vi "Read Bytes.vi"(8 "Error In":errorcluster) -> (0 "Error Out":errorcluster)   [LabVIEW 2017, in "Tests.lvlib" / "Reader.lvlib"]
uses:
  Reader.lvlib
  src/LabPack/Public/Reader/Reader.lvclass/Reader.ctl
  src/LabPack/Public/Reader/Private/Read Bytes by Value.vi
  src/LabPack/Public/Reader/Private/Handle Error.vi
  src/LabPack/Public/Reader/Public/Status/Read Status.vi
  src/LabPack/Public/Reader/Public/Status/Read Status Message.vi
  src/LabPack/Public/Reader/Public/Status/Read Is Error.vi
  src/LabPack/Public/Reader/Private/Begin Bin by Value.vi
  src/LabPack/Public/Utility/Status Code.vi
  <vilib>/Utility/error.llb/Error Cluster From Error Code.vi
  src/LabPack/Public/Reader/Private/End Bin by Value.vi
  <vilib>/addons/_JKI Toolkits/Caraya/classes/Test/Test.lvclass
  <vilib>/addons/_JKI Toolkits/Caraya/classes/Assert/Assert.lvclass
  src/LabPack/Public/Reader/Reader.lvclass
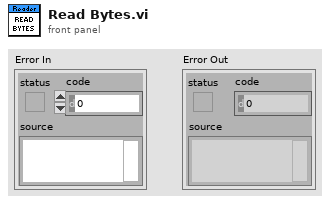
[diagram p1: front panel]
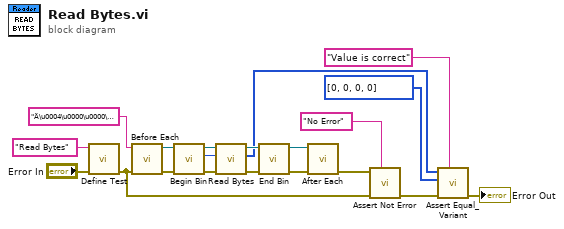
[diagram p0: block diagram]
diagram:
  n1 = call <vilib>:"Define Test.vi"("error in (no error)"="Error In", "Label (VI Title)"="Read Bytes") -> ("error out"=w17:errorcluster)  [unwired: 9 in]
  n2 = call "Before Each.vi"("Error In"=w17, "Data"="Ä\u0004\u0000\u0000\u0000\u0000") -> ("Error Out"=w9:errorcluster, "Reader"=w10:refnum<class "Reader.lvclass">)  [unwired: 8 in]
  n3 = call-poly "Begin Bin.vi"("Error In"=w9, "Reader In"=w10) -> ("Error Out"=w6:errorcluster, "Count"=w7:u32, "Reader Out"=w8:refnum<class "Reader.lvclass">)  [unwired: 7 in]
  n4 = call-poly "Read Bytes.vi"("Error In"=w6, "Count"=w7, "Reader In"=w8) -> ("Error Out"=w4:errorcluster, "Bytes"=w1:u8[], "Reader Out"=w5:refnum<class "Reader.lvclass">)  [unwired: 6 in]
  n5 = call-poly "End Bin.vi"("Error In"=w4, "Reader In"=w5) -> ("Error Out"=w3:errorcluster, "Reader Out"=w2:refnum<class "Reader.lvclass">)  [unwired: 8 in]
  n6 = call "After Each.vi"("Error In"=w3, "Reader In"=w2) -> ("Error Out"=w18:errorcluster)  [unwired: 9 in]
  n7 = call <vilib>:"Assert Not Error.vi"("Label"="No Error", "error in (no error)"=w17, "Not Error?"=w18) -> ("error out"=w16:errorcluster)  [unwired: 8 in]
  n8 = call <vilib>:"Assert Equal_Variant.vi"("Label"="Value is correct", "error in (no error)"=w16, "Y"=u8[] [0, 0, 0, 0], "X"=w1) -> ("error out"=→"Error Out":errorcluster)  [unwired: 7 in]
